vi "Initialize.vi"(8 "error in (no error)":errorcluster, 10 "DeviceName":string, 11 "HexapodController in":refnum<class "Tapedrive_ESP301.lvclass">) -> (0 "error out":errorcluster, 1 "new command(s)":string, 2 "DeviceName":string, 3 "HexapodController out":refnum<class "Tapedrive_ESP301.lvclass">)   [LabVIEW 2013, in "Tapedrive_ESP301.lvclass"]
uses:
  Tapedrive_ESP301.lvclass
  BaseDriver/BaseDriver.lvclass
  shared/CompressAndUpdate(Poly)/CompressAndUpdate(Numeric).vi
panel:
  out "Devicetype\nvariable list":string[][](array[string])
  out "Settings.devport":string
  out "Connected":bool
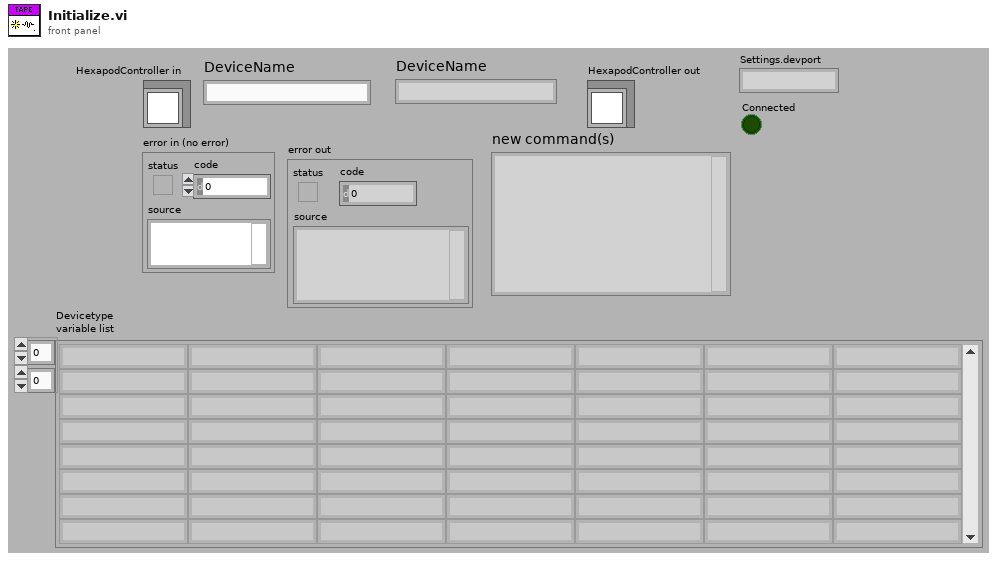
[diagram p1: front panel]
types:
  T1 = typedef "Tapedrive_ESP301.lvclass/settingsCluster_TapeDrive_TypDef.ctl" = cluster{"devport":string, "tapepos":cluster{"Value":dbl, "Min":dbl, "Max":dbl, "StepSize":dbl, "Tolerance":dbl, "ValueActual":dbl}, "status":enum16{"Not referenced", "Homing", "Moving", "Ready"}, "inmotion":T2, "forwardaxis":i16, "backwardaxis":i16, "encoderaxis":i16, "Velocity":cluster{"Axis 1":cluster{"Value":dbl, "Min":dbl, "Max":dbl, "StepSize":dbl, "Tolerance":dbl, "ValueActual":dbl}, "Axis 2":cluster{"Value":dbl, "Min":dbl, "Max":dbl, "StepSize":dbl, "Tolerance":dbl, "ValueActual":dbl}}, "Acceleration":cluster{"Axis 1":cluster{"Value":dbl, "Min":dbl, "Max":dbl, "StepSize":dbl, "Tolerance":dbl, "ValueActual":dbl}, "Axis 2":cluster{"Value":dbl, "Min":dbl, "Max":dbl, "StepSize":dbl, "Tolerance":dbl, "ValueActual":dbl}}, "Decceleration":cluster{"Axis 1":cluster{"Value":dbl, "Min":dbl, "Max":dbl, "StepSize":dbl, "Tolerance":dbl, "ValueActual":dbl}, "Axis 2":cluster{"Value":dbl, "Min":dbl, "Max":dbl, "StepSize":dbl, "Tolerance":dbl, "ValueActual":dbl}}, "MaxAcceleration":cluster{"Axis 1":cluster{"Value":dbl, "Min":dbl, "Max":dbl, "StepSize":dbl, "Tolerance":dbl, "ValueActual":dbl}, "Axis 2":cluster{"Value":dbl, "Min":dbl, "Max":dbl, "StepSize":dbl, "Tolerance":dbl, "ValueActual":dbl}}, "MaxVelocity":cluster{"Axis 1":cluster{"Value":dbl, "Min":dbl, "Max":dbl, "StepSize":dbl, "Tolerance":dbl, "ValueActual":dbl}, "Axis 2":cluster{"Value":dbl, "Min":dbl, "Max":dbl, "StepSize":dbl, "Tolerance":dbl, "ValueActual":dbl}}, "VelocityFFG":cluster{"Axis 1":cluster{"Value":dbl, "Min":dbl, "Max":dbl, "StepSize":dbl, "Tolerance":dbl, "ValueActual":dbl}, "Axis 2":cluster{"Value":dbl, "Min":dbl, "Max":dbl, "StepSize":dbl, "Tolerance":dbl, "ValueActual":dbl}}, "AccelerationFFG":cluster{"Axis 1":cluster{"Value":dbl, "Min":dbl, "Max":dbl, "StepSize":dbl, "Tolerance":dbl, "ValueActual":dbl}, "Axis 2":cluster{"Value":dbl, "Min":dbl, "Max":dbl, "StepSize":dbl, "Tolerance":dbl, "ValueActual":dbl}}, "DACoffset":cluster{"Axis 1":cluster{"Value":dbl, "Min":dbl, "Max":dbl, "StepSize":dbl, "Tolerance":dbl, "ValueActual":dbl}, "Axis 2":cluster{"Value":dbl, "Min":dbl, "Max":dbl, "StepSize":dbl, "Tolerance":dbl, "ValueActual":dbl}}, "Power":cluster{"Axis 1":T2, "Axis 2":T2}, "ReductionRatio":cluster{"Value":dbl, "Min":dbl, "Max":dbl, "StepSize":dbl, "Tolerance":dbl, "ValueActual":dbl}, "Direction":T3, "Tension":T2, "TensionVelocity":cluster{"Axis 1":cluster{"Value":dbl, "Min":dbl, "Max":dbl, "StepSize":dbl, "Tolerance":dbl, "ValueActual":dbl}, "Axis 2":cluster{"Value":dbl, "Min":dbl, "Max":dbl, "StepSize":dbl, "Tolerance":dbl, "ValueActual":dbl}}, "TensionAcceleration":cluster{"Axis 1":cluster{"Value":dbl, "Min":dbl, "Max":dbl, "StepSize":dbl, "Tolerance":dbl, "ValueActual":dbl}, "Axis 2":cluster{"Value":dbl, "Min":dbl, "Max":dbl, "StepSize":dbl, "Tolerance":dbl, "ValueActual":dbl}}, "TensionDecceleration":cluster{"Axis 1":cluster{"Value":dbl, "Min":dbl, "Max":dbl, "StepSize":dbl, "Tolerance":dbl, "ValueActual":dbl}, "Axis 2":cluster{"Value":dbl, "Min":dbl, "Max":dbl, "StepSize":dbl, "Tolerance":dbl, "ValueActual":dbl}}, "MoveVelocity":cluster{"Axis 1":cluster{"Value":dbl, "Min":dbl, "Max":dbl, "StepSize":dbl, "Tolerance":dbl, "ValueActual":dbl}, "Axis 2":cluster{"Value":dbl, "Min":dbl, "Max":dbl, "StepSize":dbl, "Tolerance":dbl, "ValueActual":dbl}}, "MoveAcceleration":cluster{"Axis 1":cluster{"Value":dbl, "Min":dbl, "Max":dbl, "StepSize":dbl, "Tolerance":dbl, "ValueActual":dbl}, "Axis 2":cluster{"Value":dbl, "Min":dbl, "Max":dbl, "StepSize":dbl, "Tolerance":dbl, "ValueActual":dbl}}, "MoveDecceleration":cluster{"Axis 1":cluster{"Value":dbl, "Min":dbl, "Max":dbl, "StepSize":dbl, "Tolerance":dbl, "ValueActual":dbl}, "Axis 2":cluster{"Value":dbl, "Min":dbl, "Max":dbl, "StepSize":dbl, "Tolerance":dbl, "ValueActual":dbl}}, "MaxStepsize":cluster{"Value":dbl, "Min":dbl, "Max":dbl, "StepSize":dbl, "Tolerance":dbl, "ValueActual":dbl}, "Stepsize":cluster{"Value":dbl, "Min":dbl, "Max":dbl, "StepSize":dbl, "Tolerance":dbl, "ValueActual":dbl}, "GoStep":T2, "StopWait":T2, "stepnum":cluster{"Value":dbl, "Min":dbl, "Max":dbl, "StepSize":dbl, "Tolerance":dbl, "ValueActual":dbl}, "MoveIfScan":T2, "HomeEncoder":T2, "Timeout":cluster{"Value":dbl, "Min":dbl, "Max":dbl, "StepSize":dbl, "Tolerance":dbl, "ValueActual":dbl}, "TapeRelax":cluster{"Value":dbl, "Min":dbl, "Max":dbl, "StepSize":dbl, "Tolerance":dbl, "ValueActual":dbl}}
  T2 = typedef "OnOffTypeDef.ctl" = enum16{"off", "on"}
  T3 = typedef "Direction.ctl" = enum16{"Forward", "Backward", "Undefined"}
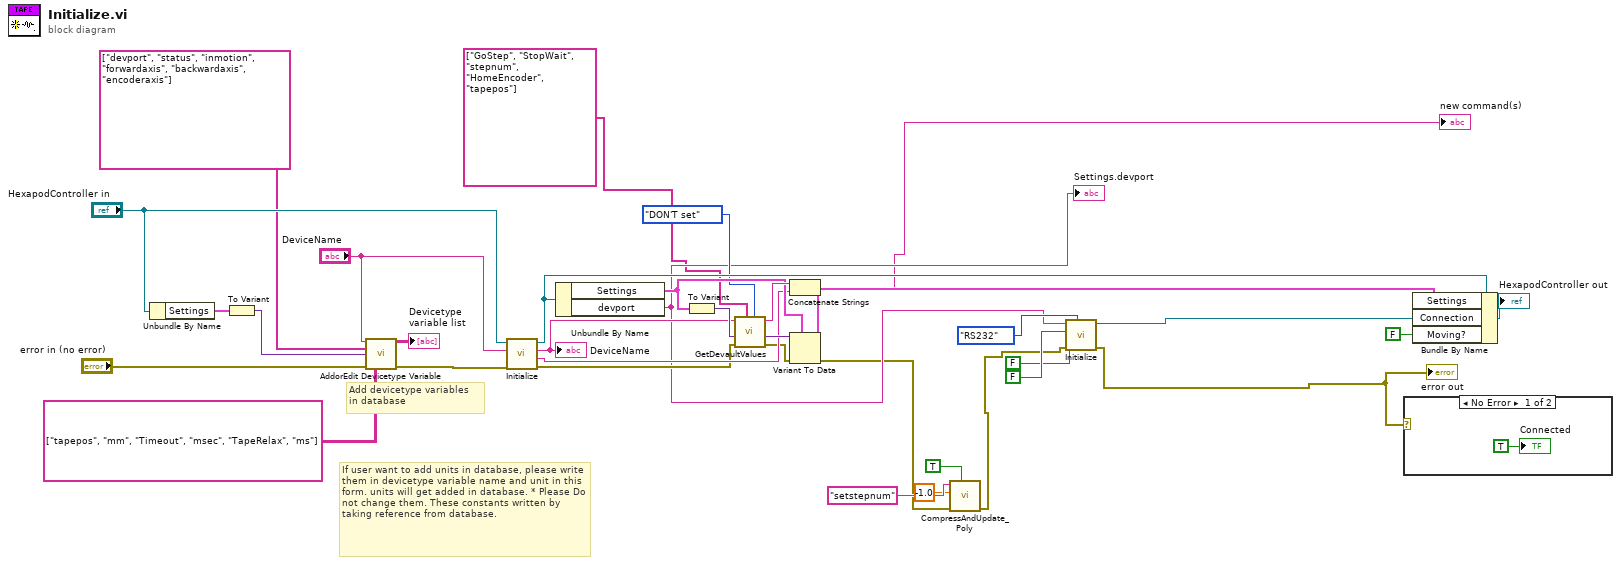
[diagram p0: block diagram]
diagram:
  # "If user want to add units in database, please write them in devicetype variable name and unit in this form. units will get added in database. * Please Do not change them. These constants written by taking reference from database."
  # "Add devicetype variables \nin database"
  n1 = Unbundle By Name("HexapodController in") -> ("Settings"=w4:T1)
  n2 = To Variant(anything=w4) -> (Variant=w3:variant)
  n3 = call "AddorEdit Devicetype Variable.vi"("Device Name"="DeviceName", "<Settings Selected elements SET=NO>"=string[] ["devport", "status", "inmotion", "forwardaxis", "backwardaxis", "encoderaxis"], "Settings variant"=w3, "error in"="error in (no error)", "Devicetype \nvariable Units"=string[][] [["tapepos", "mm"], ["Timeout", "msec"], ["TapeRelax", "ms"]] ("Devicetype \nvariable Units")) -> ("Devicetype variable list"=→"Devicetype\nvariable list":string[][], "error out"=w8:errorcluster)  [unwired: 9 in]
  n4 = call-parent <instrlib>:"Initialize.vi"("error in (no error)"=w8, "DeviceName"="DeviceName", "BaseDriver in"="HexapodController in") -> ("error out"=w25:errorcluster, "new command(s)"=w30:string, "DeviceName"=w31:string, "BaseDriver out"=w29:refnum<class "Tapedrive_ESP301.lvclass">)  [unwired: 5 in]
  "DeviceName" <- w31
  n5 = Unbundle By Name(w29) -> ("Settings"=w32:T1, "devport"=w22:string)
  "Settings.devport" <- w22
  n6 = To Variant(anything=w32) -> (Variant=w33:variant)
  n7 = call "GetDevaultValues.vi"("set or DON'T set"=enum16{"set", "DON'T set"}."DON'T set", "set following Variables (empty = all avriables)"=string[] ["GoStep", "StopWait", "stepnum", "HomeEncoder", "tapepos"], "error in (no error)"=w25, "variant"=w33, "Device Name"=w31) -> ("error out"=w24:errorcluster, "variant out"=w34:variant, "new command(s)"=w35:string)  [unwired: 4 in]
  n8 = Concatenate Strings(w35, w30) -> (→"new command(s)":string)
  n9 = Variant To Data(error in=w24, type=w32, Variant=w34) -> (data=w27:T1, error out=w13:errorcluster)
  n10 = call-poly "CompressAndUpdate_Poly.vi"("force CVT update (false)"=TRUE, "error in"=w13, "Numeric"=-1.0, "command or variable name"="setstepnum") -> ("error out"=w12:errorcluster)  [unwired: 7 in]
  n11 = call <instrlib>:"Initialize.vi"("VISA resource name"=w22, "ID Query (True)"=FALSE, "Reset (False)"=FALSE, "error in (no error)"=w12, "Serial Link (RS232)"=enum16{"RS232", "USB"}."RS232") -> ("VISA resource name out"=w11:refnum<visa-resource-name>, "error out"=w10:errorcluster)  [unwired: 4 in]
  "error out" <- w10
  n12 = case shown="No Error" w10 {
    frame No Error {
      "Connected" <- TRUE ("Connected")
    }
    frame Error {
    }
  }
  n13 = Bundle By Name(cluster=w29, "Settings"=w27, "Connection"=w11, "Moving?"=FALSE ("Wait for Step")) -> (→"HexapodController out":refnum<class "Tapedrive_ESP301.lvclass">)
